vi "Initialize.vi"(8 "error in (no error)":errorcluster, 11 "7-zip Wrapper in":refnum<class "7-zip Wrapper.lvclass">) -> (0 "error out":errorcluster, 3 "7-zip Wrapper out":refnum<class "7-zip Wrapper.lvclass">)   [LabVIEW 2020, in "7-zip Wrapper.lvclass"]
doc: "This is a factory method that will encapsulate all complexity needed to start sending the console commands. Initially the required steps you must set the Application Name and the Working directory parameters. If you do not set those values, the Application Name will be empty and the working directory will be C:. It will also pass the command \"dir\" wihtout any options."
uses:
  7-zip Wrapper.lvclass
  C:/Users/fflores/Documents/GitHub Projects/LabVIEW-CLI-Wrapper/Console Wrapper/Console Wrapper.lvclass
  Console Wrapper/Console Wrapper.lvclass/Console Wrapper.ctl
  Console Wrapper/Write Application Name.vi
  Console Wrapper/Write Working Directory.vi
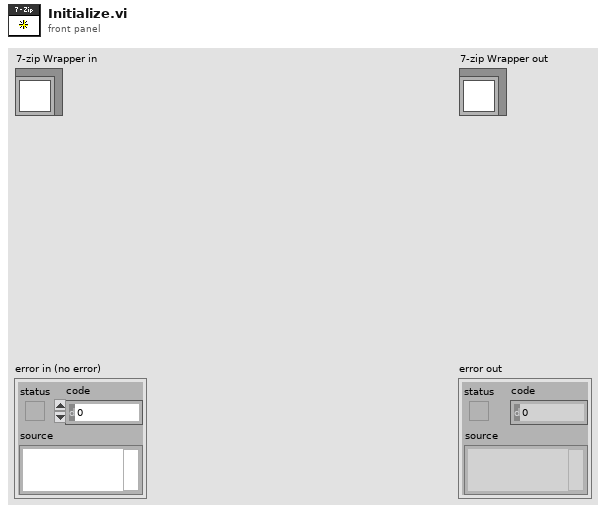
[diagram p1: front panel]
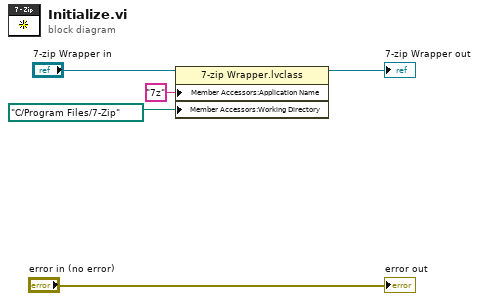
[diagram p0: block diagram]
diagram:
  n1 = property class="7-zip Wrapper.lvclass"(reference="7-zip Wrapper in", "Member Accessors:Application Name"="7z" ("Application Name"), "Member Accessors:Working Directory"=path "C:/Program Files/7-Zip" ("working directory")) -> (reference out=→"7-zip Wrapper out":refnum<class "7-zip Wrapper.lvclass">)  [unwired: 1 in, 1 out]
  "error out" <- "error in (no error)"
